vi "Instrument Configure.vi"(0 "RFSG Session In":refnum<k15>, 5 "SG Configuration":T1={"Reference Clock Source"="OnboardClock", "Carrier Frequency (Hz)"=1000000000.0, "DUT Average Input Power (dBm)"=-20.0, "External Attenuation (dB)"=0.0, "Marker 0 Export Terminal"="", "Share LO  SG->SA"=FALSE} {"Carrier Frequency (Hz)" format="%#_6p"}, 11 "error in (no error)":errorcluster) -> (4 "RFSG Session Out":refnum<k15>, 15 "error out":errorcluster)   [LabVIEW 2018, in "SG.lvlib"]
uses:
  SG.lvlib
  Typedefs/Instrument Configuration.ctl
  <instrlib>/niRFSG/niRFSG.llb/niRFSG Ref Clock Sources.ctl
  <instrlib>/niRFSG/niRFSG.llb/niRFSG Trigger Terminals.ctl
  <instrlib>/niRFSG/niRFSG.llb/niRFSG Signal Names.ctl
  <instrlib>/niRFSG/niRFSG.llb/niRFSG Signal Identifiers.ctl
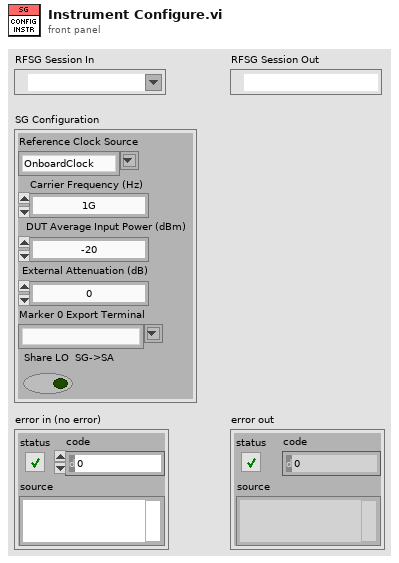
[diagram p1: front panel]
types:
  T1 = typedef "SG.lvlib/Instrument Configuration.ctl" = cluster{"Reference Clock Source":T2, "Carrier Frequency (Hz)":dbl, "DUT Average Input Power (dBm)":dbl, "External Attenuation (dB)":dbl, "Marker 0 Export Terminal":T3, "Share LO  SG->SA":bool}
  T2 = typedef "niRFSG Ref Clock Sources.ctl" = string
  T3 = typedef "niRFSG Trigger Terminals.ctl" = string
  T4 = typedef "niRFSG Signal Identifiers.ctl" = string
  T5 = typedef "niRFSG Signal Names.ctl" = i32
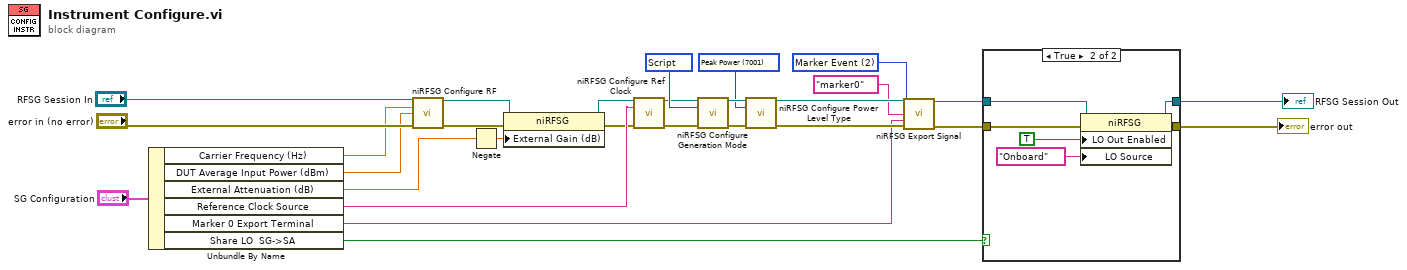
[diagram p0: block diagram]
diagram:
  w19 = T5 2 items=["Start Trigger", "Script Trigger", "Marker Event", "Ref Clock", "Started Event", "Done Event", "Configuration List Step Trigger", "Configuration Settled Event"] ("signal")
  w12 = 7001 items=["Average Power"=7000, "Peak Power"=7001] ("power level type")
  w24 = 1002 items=["CW"=1000, "Arb Waveform"=1001, "Script"=1002] ("generation mode")
  n1 = Unbundle By Name("SG Configuration") -> ("Carrier Frequency (Hz)"=w7:dbl, "DUT Average Input Power (dBm)"=w6:dbl, "External Attenuation (dB)"=w2:dbl, "Reference Clock Source"=w23:T2, "Marker 0 Export Terminal"=w21:T3, "Share LO  SG->SA"=w17:bool)
  n2 = call <instrlib>:"niRFSG Configure RF.vi"("instrument handle"="RFSG Session In", "frequency (Hz)"=w7, "power level (dBm)"=w6, "error in"="error in (no error)") -> ("instrument handle out"=w4:refnum<k15>, "error out"=w9:errorcluster)  [unwired: 10 in]
  n3 = Negate(x=w2) -> (-x=w1:dbl)
  n4 = property class="niRFSG"(reference=w4, error in=w9, "External Gain (dB)"=w1) -> (reference out=w3:refnum<k15>, error out=w5:errorcluster)
  n5 = call <instrlib>:"niRFSG Configure Ref Clock.vi"("instrument handle"=w3, "ref clock source"=w23, "error in"=w5) -> ("instrument handle out"=w14:refnum<k15>, "error out"=w13:errorcluster)  [unwired: 11 in]
  n6 = call <instrlib>:"niRFSG Configure Generation Mode.vi"("instrument handle"=w14, "generation mode"=w24, "error in"=w13) -> ("instrument handle out"=w28:refnum<k15>, "error out"=w27:errorcluster)  [unwired: 11 in]
  n7 = call <instrlib>:"niRFSG Configure Power Level Type.vi"("instrument handle"=w28, "power level type"=w12, "error in"=w27) -> ("instrument handle out"=w20:refnum<k15>, "error out"=w26:errorcluster)  [unwired: 11 in]
  n8 = call <instrlib>:"niRFSG Export Signal.vi"("instrument handle"=w20, "signal"=w19, "signal identifier"=T4 "marker0", "output terminal"=w21, "error in"=w26) -> ("instrument handle out"=w10:refnum<k15>, "error out"=w11:errorcluster)  [unwired: 9 in]
  n9 = case shown="True" w17 {
    tunnel: w11 -> [w29 w36]
    tunnel: w10 -> [w30 w35]
    tunnel: [w29 w34] -> w16
    tunnel: [w30 w33] -> w15
    frame False {
    }
    frame True {
      n10 = property class="niRFSG"(reference=w35, error in=w36, "LO Out Enabled"=TRUE ("RF:LO Out Enabled"), "LO Source"="Onboard" ("Device Specific:Vector Signal Transceiver:Signal Path:LO Source")) -> (reference out=w33:refnum<k15>, error out=w34:errorcluster)
    }
  }
  "error out" <- w16
  "RFSG Session Out" <- w15
